vi "Problems.vi"(8 "Error in":errorcluster, 11 "Problems":refnum<k24>) -> (0 "Error out":errorcluster)   [LabVIEW 2016]
doc: "Generates an error, if the problems (eg. as a result of an assign function) contain any errors.\nGenerates a warning, if the problems contain any warning but no error."
uses:
  C:/Users/CL/Desktop/ZcDAQprj0811/ZcDAQprj/Modules/DAQ-Device/Hardware Drivers/QX/HBM LabVIEW Driver/DLLs/Hbm.Api.Common.dll
  DLLs/Hbm.Api.Common.dll
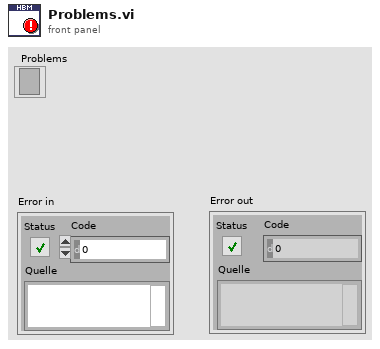
[diagram p1: front panel]
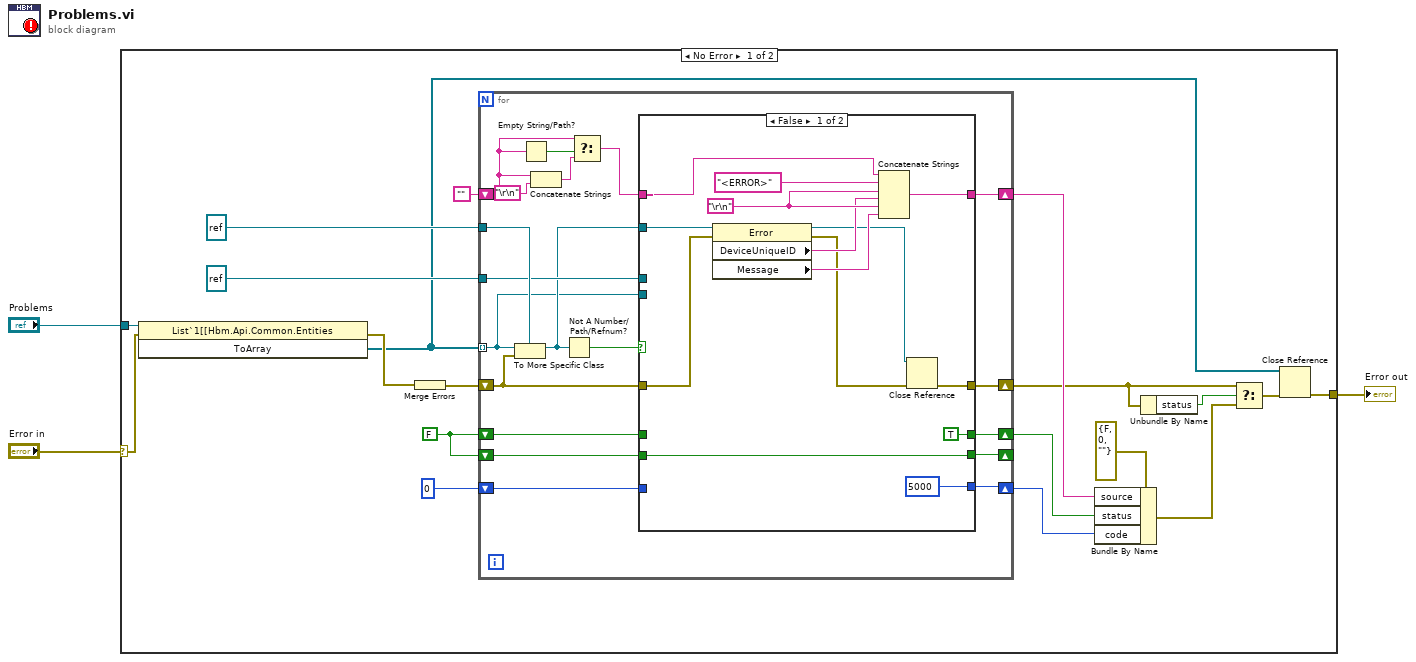
[diagram p0: block diagram]
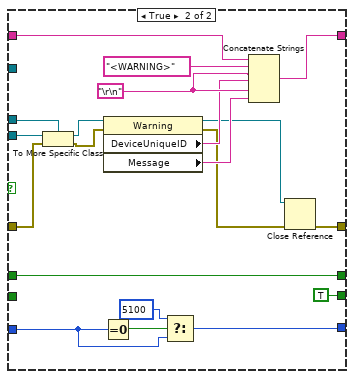
[diagram p2: hidden frame]
diagram:
  n1 = case shown="No Error" "Error in" {
    selector: "Error in" -> [w10 w76]
    tunnel: "Problems" -> [w22 _]
    tunnel: [w4 w76] -> w3
    frame No Error {
      w19 = FALSE
      n2 = invoke on="Methodenknoten" class="List`1[[Hbm.Api.Common.Entities" method="ToArray"(reference=w22, error in=w10) -> (error out=w21:errorcluster, "ToArray"=w5:refnum<k24>[])  [unwired: 1 in, 1 out]
      n3 = Merge Errors(w21) -> (w20:errorcluster)
      n4 = for {
        tunnel: w5 -> [w27] mode=indexing
        tunnel: refnum<k24> refnum (".NET (Referenz)") -> [w40]
        tunnel: refnum<k24> refnum (".NET (Referenz)") -> [w39]
        shift-right: [w38] -> w9
        shift-left: w20 -> [w23]
        shift-right: [w36] -> w12
        shift-left: w19 -> [w37]
        shift-right: [w35] -> _
        shift-left: w19 -> [w34]
        shift-right: [w33] -> w13
        shift-left: "" -> [w26]
        shift-right: [w29] -> w11
        shift-left: 0 ("t") -> [w30]
        n5 = To More Specific Class(target class=w40, reference=w27, error in=w23) -> (specific class reference=w28:refnum<k24>)  [unwired: 1 out]
        n6 = Empty String/Path?(string/path=w26) -> (empty?=w32:bool)
        n7 = Concatenate Strings(w26, "\r\n") -> (w24:string)
        n8 = Not A Number/Path/Refnum?(number/path/refnum=w28) -> (NaN/Path/Refnum?=w41:bool)
        n9 = Select(t=w26, s=w32, f=w24) -> (s? t:f=w31:string)
        n10 = case shown="False" w41 {
          tunnel: w28 -> [w54 _]
          tunnel: w39 -> [_ w63]
          tunnel: [w53 w74] -> w33
          tunnel: w23 -> [w52 w59]
          tunnel: [w44 w58] -> w38
          tunnel: w37 -> [_ w73]
          tunnel: w34 -> [w51 _]
          tunnel: [TRUE w73] -> w36
          tunnel: [w51 TRUE] -> w35
          tunnel: w31 -> [w46 w68]
          tunnel: w30 -> [_ w65]
          tunnel: [5000 ("t") w64] -> w29
          tunnel: w27 -> [_ w60]
          frame False {
            w49 = "\r\n"
            n11 = property class="Error"(reference=w54, error in=w52) -> (reference out=w42:refnum<k24>, error out=w43:errorcluster, "DeviceUniqueID"=w48:string, "Message"=w47:string)
            n12 = Concatenate Strings(w46, "<ERROR>" ("Element"), w49, w48, w49, w47) -> (w53:string)
            n13 = Close Reference(reference=w42, error in (no error)=w43) -> (error out=w44:errorcluster)
          }
          frame True {
            w71 = "\r\n"
            n14 = To More Specific Class(target class=w63, reference=w60, error in=w59) -> (specific class reference=w62:refnum<k24>, error out=w61:errorcluster)
            n15 = Equal To 0?(x=w65) -> (x = 0?=w66:bool)
            n16 = property class="Warning"(reference=w62, error in=w61) -> (reference out=w56:refnum<k24>, error out=w57:errorcluster, "DeviceUniqueID"=w70:string, "Message"=w69:string)
            n17 = Select(t=5100, s=w66, f=w65) -> (s? t:f=w64:i32)
            n18 = Concatenate Strings(w68, "<WARNING>" ("Element"), w71, w70, w71, w69) -> (w74:string)
            n19 = Close Reference(reference=w56, error in (no error)=w57) -> (error out=w58:errorcluster)
          }
        }
      }
      n20 = Bundle By Name(cluster=errorcluster {"status"=FALSE, "code"=0, "source"=""} ("error out"), "source"=w13, "status"=w12, "code"=w11) -> (w16:errorcluster)
      n21 = Unbundle By Name(w9) -> ("status"=w15:bool)
      n22 = Select(t=w9, s=w15, f=w16) -> (s? t:f=w6:errorcluster)
      n23 = Close Reference(reference=w5, error in (no error)=w6) -> (error out=w4:errorcluster)
    }
    frame Error {
    }
  }
  "Error out" <- w3
